vi "Config ACTION.vi"(8 "error in (no error)":errorcluster, 11 "Scale Calibration in":refnum<class "Scale Calibration.lvclass">) -> (0 "error out":errorcluster, 3 "Scale Calibration out":refnum<class "Scale Calibration.lvclass">)   [LabVIEW 2014, in "SeqLoop.lvlib" / "STEP Classes.lvlib" / "Scale Calibration.lvclass"]
uses:
  Scale Calibration.lvclass
  Scale Calibration.lvclass/Scale Calibration.ctl
panel:
  in  "Cancel":bool
  in  "Save":bool
  in  "Calibrar Balanzas?":bool
  # "Dispositivos de Hardware para relevamiento"
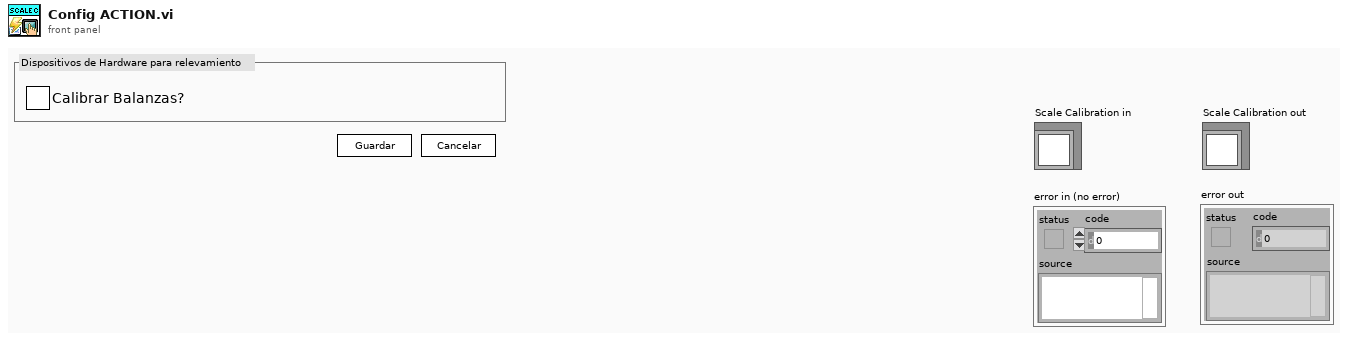
[diagram p1: front panel]
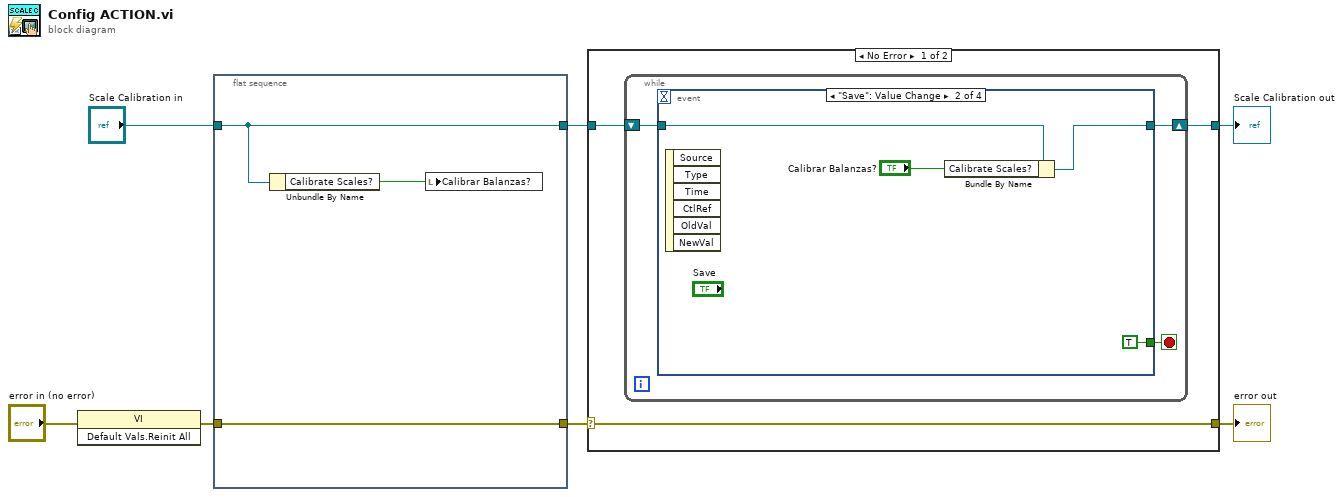
[diagram p0: block diagram]
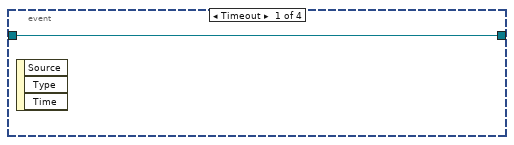
[diagram p2: hidden frame]
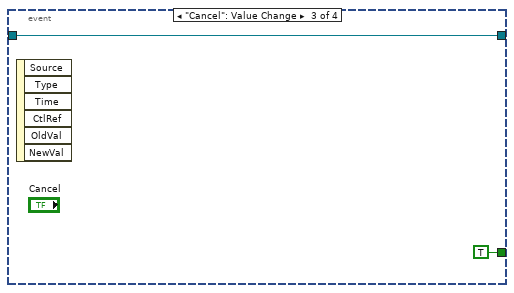
[diagram p3: hidden frame]
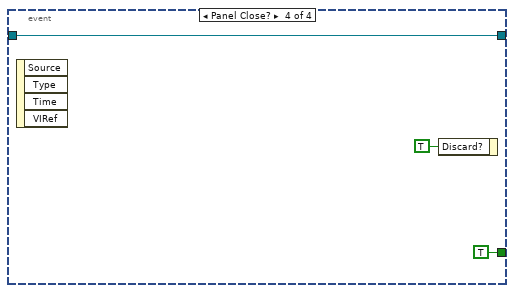
[diagram p4: hidden frame]
diagram:
  n1 = invoke class="VI" method="Default Vals.Reinit All"(error in="error in (no error)") -> (error out=w6:errorcluster)  [unwired: 2 in, 2 out]
  n2 = flat-sequence {
    tunnel: "Scale Calibration in" -> [w10]
    tunnel: [w9] -> w7
    tunnel: w6 -> [w9]
    tunnel: [w10] -> w5
    frame #0 {
      n3 = Unbundle By Name(w10) -> ("Calibrate Scales?"=w8:bool)
      n4 = local write "Calibrar Balanzas?"(w8) -> ()
    }
  }
  n5 = case shown="No Error" w7 {
    selector: w7 -> [w13 w28]
    tunnel: [w13 w28] -> w1
    tunnel: [w11 w27] -> w2
    tunnel: w5 -> [w12 w27]
    frame No Error {
      n6 = while {
        shift-right: [w15] -> w11
        shift-left: w12 -> [w16]
        stop <- w14 stop-if-true
        n7 = event shown="[1] \"Save\": Value Change" {
          selector: _ -> [_ _ _ _]
          dyn-events: _ -> [_ _ _ _]
          timeout: _ -> [_ _ _ _]
          tunnel: w16 -> [w17 w20 w23 w26]
          tunnel: [w17 w19 w23 w26] -> w15
          tunnel: [_ TRUE TRUE TRUE] -> w14
          event Timeout {
            n8 = event-data() -> ()  [unwired: 1 in, 3 out]
          }
          event "Save": Value Change {
            n9 = event-data() -> ()  [unwired: 1 in, 6 out]
            n10 = Bundle By Name(cluster=w20, "Calibrate Scales?"="Calibrar Balanzas?") -> (w19:refnum<class "Scale Calibration.lvclass">)
          }
          event "Cancel": Value Change {
            n11 = event-data() -> ()  [unwired: 1 in, 6 out]
          }
          event Panel Close? {
            n12 = event-data() -> ()  [unwired: 1 in, 4 out]
            n13 = event-data("Discard?"=TRUE) -> ()  [unwired: 1 in, 1 out]
          }
        }
      }
    }
    frame Error {
    }
  }
  "error out" <- w1
  "Scale Calibration out" <- w2
